vi "Cleanup.vi"(8 "error in (no error)":errorcluster, 11 "DeviceListPanel in":refnum<class "DeviceListPanel.lvclass">) -> (0 "error out":errorcluster)   [LabVIEW 2020, in "PicoG-App.lvlib" / "DeviceListPanel.lvclass"]
uses:
  DeviceListPanel.lvclass
  DeviceListPanel.lvclass/DeviceListPanel.ctl
  <vilib>/IlluminatedG/IG OOPanel/OOPanel/Panel/Panel.lvclass
  <vilib>/IlluminatedG/IG OOPanel/OOPanel/ArrayManager/ArrayManager.lvclass
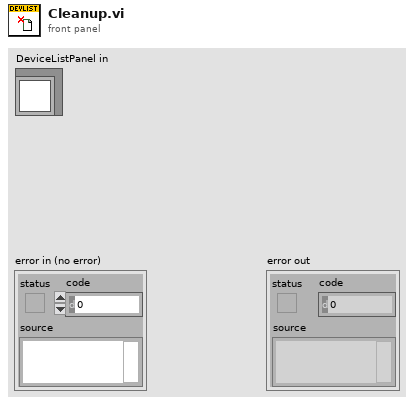
[diagram p1: front panel]
types:
  T1 = typedef "PicoG-App.lvlib/DeviceListPanel.lvclass/Inbound Events.ctl" = cluster{"Add Device":refnum<user-event>, "Select Device":refnum<user-event>, "Remove Device":refnum<user-event>, "Refresh Device":refnum<user-event>}
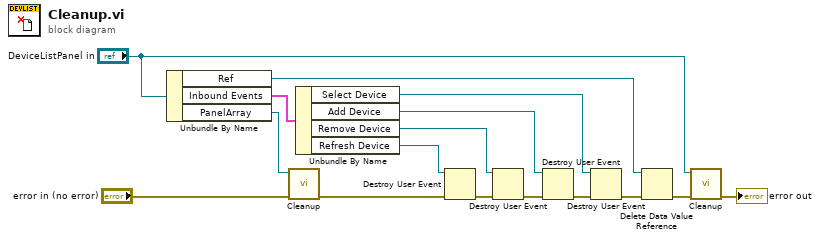
[diagram p0: block diagram]
diagram:
  n1 = Unbundle By Name("DeviceListPanel in") -> ("Ref"=w14:refnum<data-value>, "Inbound Events"=w15:T1, "PanelArray"=w16:refnum<class "ArrayManager.lvclass">)
  n2 = call <vilib>:"Cleanup.vi"("error in (no error)"="error in (no error)", "PanelArray in"=w16) -> ("error out"=w1:errorcluster)  [unwired: 9 in]
  n3 = Unbundle By Name(w15) -> ("Select Device"=w6:refnum<user-event>, "Add Device"=w13:refnum<user-event>, "Remove Device"=w3:refnum<user-event>, "Refresh Device"=w2:refnum<user-event>)
  n4 = Destroy User Event(user event=w2, error in=w1) -> (error out=w5:errorcluster)
  n5 = Destroy User Event(user event=w3, error in=w5) -> (error out=w4:errorcluster)
  n6 = Destroy User Event(user event=w13, error in=w4) -> (error out=w12:errorcluster)
  n7 = Destroy User Event(user event=w6, error in=w12) -> (error out=w11:errorcluster)
  n8 = Delete Data Value Reference(data value reference=w14, error in=w11) -> (error out=w10:errorcluster)  [unwired: 1 out]
  n9 = call-parent <vilib>:"Cleanup.vi"("error in (no error)"=w10, "Panel in"="DeviceListPanel in") -> ("error out"=→"error out":errorcluster)  [unwired: 9 in]
